vi "Done Or Abort.vi"(3 "error in (no error)":errorcluster, 4 "timeout":i32=200, 6 "MCL State In":refnum<queue>) -> (0 "error out":errorcluster, 1 "MCL State":T1, 2 "MCL State Out":refnum<queue>)   [LabVIEW 2013]
uses:
  MCL Done Or Abort.ctl
  MixedMode/MCL States.ctl
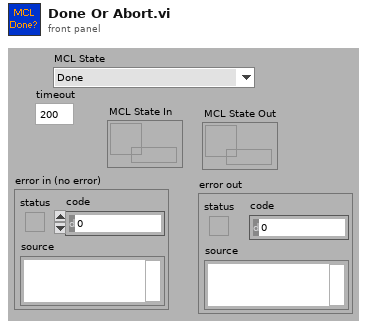
[diagram p1: front panel]
types:
  T1 = typedef "MCL Done Or Abort.ctl" = enum16{"Done", "Abort", "Still Running"}
  T2 = typedef "MCL States.ctl" = enum16{"MCL Idle", "MCL Ramping", "MCL Holding", "MCL Aborting", "MCL Done", "MCL NOP"}
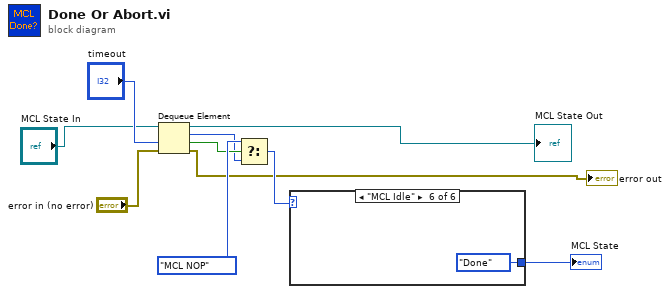
[diagram p0: block diagram]
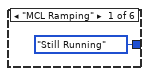
[diagram p2: hidden frame]
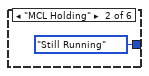
[diagram p3: hidden frame]
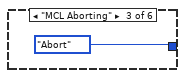
[diagram p4: hidden frame]
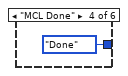
[diagram p5: hidden frame]
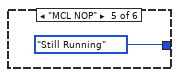
[diagram p6: hidden frame]
diagram:
  n1 = Dequeue Element(queue="MCL State In", timeout in ms (-1)="timeout", error in (no error)="error in (no error)") -> (queue out=→"MCL State Out":refnum<queue>, element=w3:T2, timed out?=w9:bool, error out=→"error out":errorcluster)
  n2 = Select(t=MCL_States."MCL NOP", s=w9, f=w3) -> (s? t:f=w8:T2)
  n3 = case shown="\"MCL Idle\"" w8 {
    tunnel: [MCL_Done_Or_Abort."Still Running" ("MCL State") MCL_Done_Or_Abort."Still Running" ("MCL State") MCL_Done_Or_Abort."Abort" ("MCL State") MCL_Done_Or_Abort."Done" ("MCL State") MCL_Done_Or_Abort."Still Running" ("MCL State") MCL_Done_Or_Abort."Done" ("MCL State")] -> w4
    frame "MCL Ramping" {
    }
    frame "MCL Holding" {
    }
    frame "MCL Aborting" {
    }
    frame "MCL Done" {
    }
    frame "MCL NOP" {
    }
    frame "MCL Idle" {
    }
  }
  "MCL State" <- w4
